vi "Dialog-SeriesName.vi"() -> (0 "String":string, 3 "Anulowane?":bool)   [LabVIEW 2019]
panel:
  in  "Nazwa serii pomiarowej":string
  in  "OK":bool
  in  "Anuluj":bool
  # "Wpisz nazwê serii pomiarowej"
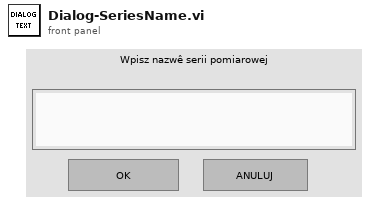
[diagram p1: front panel]
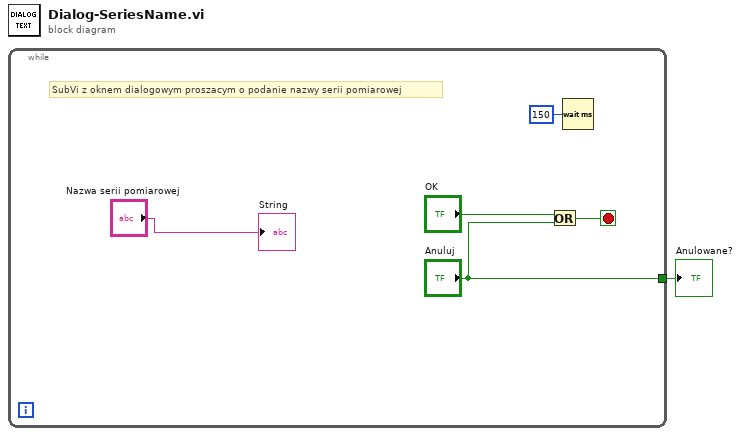
[diagram p0: block diagram]
diagram:
  n1 = while {
    tunnel: ["Anuluj"] -> w1
    stop <- w5 stop-if-true
    # "SubVi z oknem dialogowym proszacym o podanie nazwy serii pomiarowej"
    n2 = Or(x="OK", y="Anuluj") -> (x .or. y?=w5:bool)
    n3 = Wait (ms)(milliseconds to wait=u32 150) -> ()  [unwired: 1 out]
    "String" <- "Nazwa serii pomiarowej"
  }
  "Anulowane?" <- w1
